vi "Check_Server.vi"(3 "timeout ms (60000)":i32, 5 "address":string) -> (1 "OK":bool)   [LabVIEW 2016]
panel:
  out "error out":errorcluster
  out "connection ID":refnum<k5>
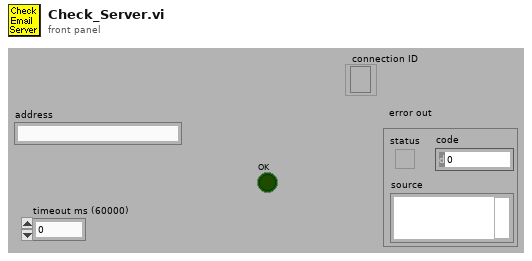
[diagram p1: front panel]
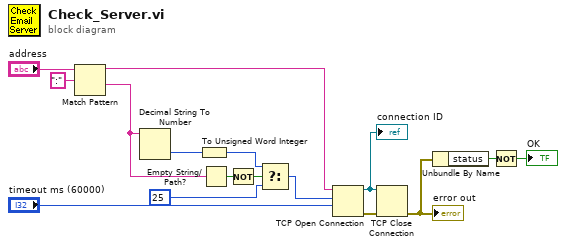
[diagram p0: block diagram]
diagram:
  n1 = Match Pattern(string="address", regular expression=":") -> (before substring=w8:string, after substring=w5:string)  [unwired: 1 in, 2 out]
  n2 = Decimal String To Number(string=w5) -> (number=w4:i32)  [unwired: 2 in, 1 out]
  n3 = To Unsigned Word Integer(number=w4) -> (unsigned 16bit integer=w2:u16)
  n4 = Empty String/Path?(string/path=w5) -> (empty?=w6:bool)
  n5 = Not(x=w6) -> (.not. x?=w7:bool)
  n6 = Select(t=w2, s=w7, f=u16 25 ("remote port")) -> (s? t:f=w1:u16)
  n7 = TCP Open Connection(address=w8, remote port or service name=w1, timeout ms (60000)="timeout ms (60000)") -> (connection ID=w11:refnum<k5>, error out=w15:errorcluster)  [unwired: 1 in, 1 out]
  "connection ID" <- w11
  n8 = TCP Close Connection(connection ID=w11, error in (no error)=w15) -> (error out=w14:errorcluster)  [unwired: 2 out]
  "error out" <- w14
  n9 = Unbundle By Name(w14) -> ("status"=w13:bool)
  n10 = Not(x=w13) -> (.not. x?=→"OK":bool)
